vi "Configure Averaging.vi"(6 "Averaging Count (16)":i32=16 format="%^#_9g", 7 "Enable Averaging Restart (Disable)":bool, 8 "error in (no error)":errorcluster, 9 "Enable Averaging (Disable)":bool, 10 "Measurement Type (6: Phase Noise)":u16(ring)=6 items=["AM Noise"=1, "Baseband Noise"=2, "Freq/Power"=3, "Spectrum"=4, "Transient"=5, "Phase Noise"=6, "User"=7], 11 "VISA resource name":refnum<visa-resource-name>) -> (0 "error out":errorcluster, 3 "VISA resource name out":refnum<visa-resource-name>)   [LabVIEW 2011, in "Agilent E5052X.lvlib"]
doc: "Sets the averaging function for all measurements except the User measurement. The averaging function averages a number of measurements set by the \"Averaging Count\" control and displays the final result."
uses:
  Agilent E5052X.lvlib
panel:
  # "Averaging Settings"
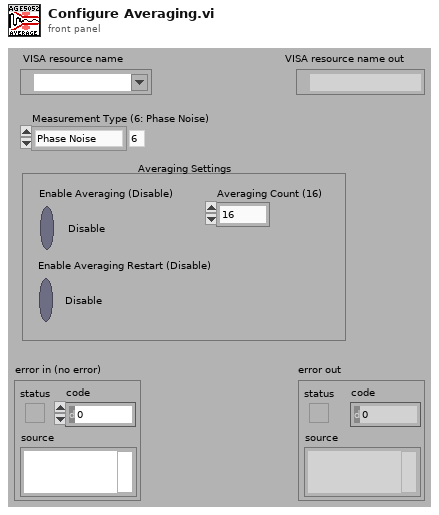
[diagram p1: front panel]
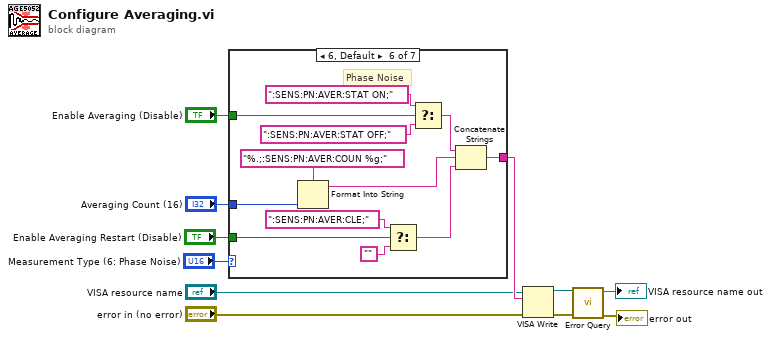
[diagram p0: block diagram]
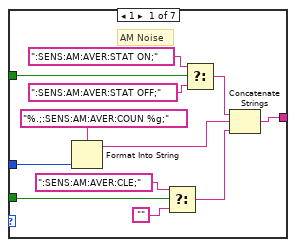
[diagram p2: hidden frame]
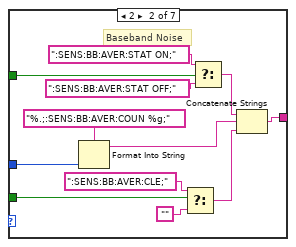
[diagram p3: hidden frame]
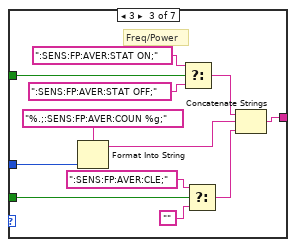
[diagram p4: hidden frame]
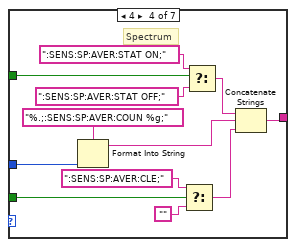
[diagram p5: hidden frame]
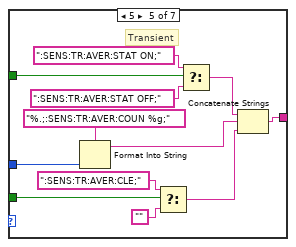
[diagram p6: hidden frame]
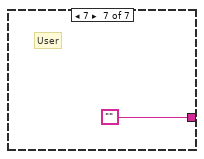
[diagram p7: hidden frame]
diagram:
  n1 = case shown="6, Default" "Measurement Type (6: Phase Noise)" {
    tunnel: "Enable Averaging (Disable)" -> [w16 w30 w41 w53 w64 w77 _]
    tunnel: "Averaging Count (16)" -> [w23 w33 w45 w57 w69 w81 _]
    tunnel: [w20 w32 w44 w56 w68 w80 ""] -> w9
    tunnel: "Enable Averaging Restart (Disable)" -> [w13 w26 w36 w49 w61 w73 _]
    frame 1 {
      # "AM Noise"
      n2 = Format Into String(format string="%.;:SENS:AM:AVER:COUN %g;", w23) -> (resulting string=w21:string)  [unwired: 2 in, 1 out]
      n3 = Select(t=":SENS:AM:AVER:CLE;", s=w13, f="") -> (s? t:f=w12:string)
      n4 = Select(t=":SENS:AM:AVER:STAT ON;", s=w16, f=":SENS:AM:AVER:STAT OFF;") -> (s? t:f=w17:string)
      n5 = Concatenate Strings(w17, w21, w12) -> (w20:string)
    }
    frame 2 {
      # "Baseband Noise"
      n6 = Format Into String(format string="%.;:SENS:BB:AVER:COUN %g;", w33) -> (resulting string=w34:string)  [unwired: 2 in, 1 out]
      n7 = Select(t=":SENS:BB:AVER:CLE;", s=w26, f="") -> (s? t:f=w25:string)
      n8 = Select(t=":SENS:BB:AVER:STAT ON;", s=w30, f=":SENS:BB:AVER:STAT OFF;") -> (s? t:f=w29:string)
      n9 = Concatenate Strings(w29, w34, w25) -> (w32:string)
    }
    frame 3 {
      # "Freq/Power"
      n10 = Format Into String(format string="%.;:SENS:FP:AVER:COUN %g;", w45) -> (resulting string=w46:string)  [unwired: 2 in, 1 out]
      n11 = Select(t=":SENS:FP:AVER:STAT ON;", s=w41, f=":SENS:FP:AVER:STAT OFF;") -> (s? t:f=w40:string)
      n12 = Select(t=":SENS:FP:AVER:CLE;", s=w36, f="") -> (s? t:f=w37:string)
      n13 = Concatenate Strings(w40, w46, w37) -> (w44:string)
    }
    frame 4 {
      # "Spectrum"
      n14 = Format Into String(format string="%.;:SENS:SP:AVER:COUN %g;", w57) -> (resulting string=w58:string)  [unwired: 2 in, 1 out]
      n15 = Select(t=":SENS:SP:AVER:CLE;", s=w49, f="") -> (s? t:f=w48:string)
      n16 = Select(t=":SENS:SP:AVER:STAT ON;", s=w53, f=":SENS:SP:AVER:STAT OFF;") -> (s? t:f=w52:string)
      n17 = Concatenate Strings(w52, w58, w48) -> (w56:string)
    }
    frame 5 {
      # "Transient"
      n18 = Format Into String(format string="%.;:SENS:TR:AVER:COUN %g;", w69) -> (resulting string=w70:string)  [unwired: 2 in, 1 out]
      n19 = Select(t=":SENS:TR:AVER:CLE;", s=w61, f="") -> (s? t:f=w60:string)
      n20 = Select(t=":SENS:TR:AVER:STAT ON;", s=w64, f=":SENS:TR:AVER:STAT OFF;") -> (s? t:f=w65:string)
      n21 = Concatenate Strings(w65, w70, w60) -> (w68:string)
    }
    frame 6, Default {
      # "Phase Noise"
      n22 = Format Into String(format string="%.;:SENS:PN:AVER:COUN %g;", w81) -> (resulting string=w82:string)  [unwired: 2 in, 1 out]
      n23 = Select(t=":SENS:PN:AVER:CLE;", s=w73, f="") -> (s? t:f=w72:string)
      n24 = Select(t=":SENS:PN:AVER:STAT ON;", s=w77, f=":SENS:PN:AVER:STAT OFF;") -> (s? t:f=w76:string)
      n25 = Concatenate Strings(w76, w82, w72) -> (w80:string)
    }
    frame 7 {
      # "User"
    }
  }
  n26 = VISA Write(VISA resource name="VISA resource name", write buffer=w9, error in (no error)="error in (no error)") -> (VISA resource name out=w8:refnum<visa-resource-name>, error out=w7:errorcluster)  [unwired: 1 out]
  n27 = call "Error Query.vi"("error in (no error)"=w7, "VISA resource name"=w8) -> ("error out"=→"error out":errorcluster, "VISA resource name out"=→"VISA resource name out":refnum<visa-resource-name>)  [unwired: 6 in, 2 out]
